vi "normalize.vi"(8 "error in":errorcluster caption="entrée d'erreur", 9 "X":string[][](array[string]), 10 "Type X":T1(ring), 11 "normalize":T3={"norm"="l2", "axis"=1, "copy"=TRUE, "Returns"="X"}) -> (0 "error out":errorcluster caption="sortie d'erreur", 3 "Data":T2)   [LabVIEW 2020]
uses:
  normalize.lvclass
panel:
  out "normalize.lvclass":refnum<class "normalize.lvclass">
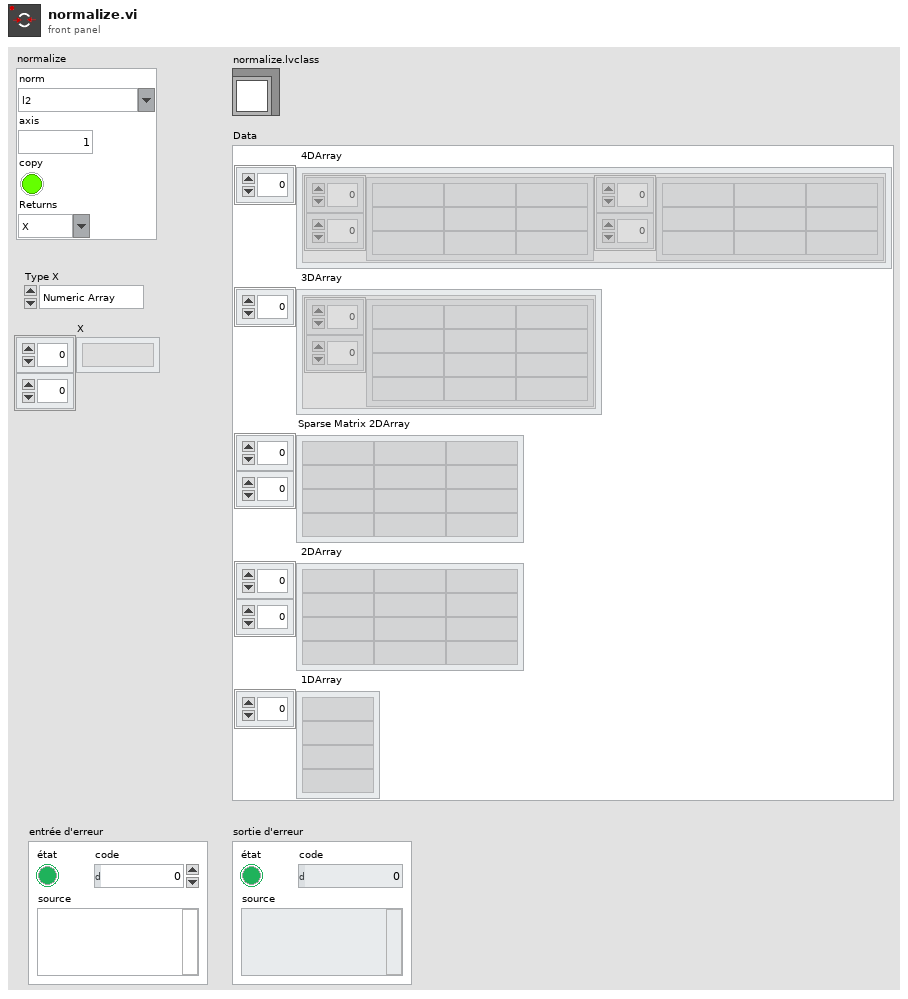
[diagram p1: front panel]
types:
  T1 = enum16{"Numeric Array", "String Array", "Sparse"}
  T2 = cluster{" 4DArray":cluster{"1":string[][], "2":string[][]}[], " 3DArray":cluster{"Tableau":string[][]}[], "Sparse Matrix 2DArray":string[][], " 2DArray":string[][], " 1DArray":string[]}
  T3 = cluster{"norm":string, "axis":i32, "copy":bool, "Returns":string}
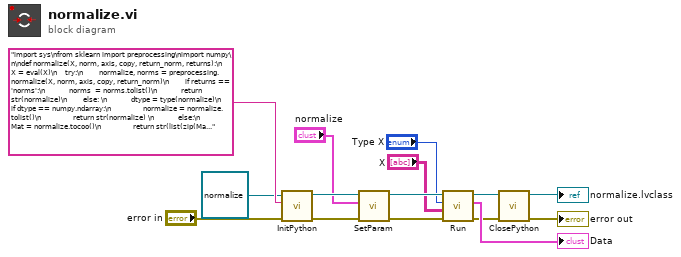
[diagram p0: block diagram]
diagram:
  n1 = call-dynamic "InitPython.vi"("error in (no error)"="error in", "Python Instruction"="import sys\nfrom sklearn import preprocessing\nimport numpy\n\ndef normalize(X, norm, axis, copy, return_norm, returns):\n    X = eval(X)\n    try:\n        normalize, norms = preprocessing.normalize(X, norm, axis, copy, return_norm)\n        if returns == 'norms':\n            norms  = norms.tolist()\n            return str(normalize)\n        else: \n            dtype = type(normalize)\n            if dtype == numpy.ndarray:\n                normalize = normalize.tolist()\n                return str(normalize) \n            else:\n                Mat = normalize.tocoo()\n                return str(list(zip(Mat.row, Mat.col, Mat.data)))\n    except:\n        erreur = sys.exc_info()\n        typerr = u\"%s\" % (erreur[0])\n        typerr = typerr[typerr.find(\"'\")+1:typerr.rfind(\"'\")]\n        msgerr = u\"%s\" % (erreur[1])\n        message = str('/!\\\\ {0} : {1}'. format(typerr,msgerr))\n        return message", "Scikit-learn en entrée"=refnum<class "normalize.lvclass"> refnum ("normalize.lvclass")) -> ("error out"=w10:errorcluster, "Scikit-learn en sortie"=w11:refnum<class "normalize.lvclass">)  [unwired: 7 in]
  n2 = call-dynamic "SetParam.vi"("error in (no error)"=w10, "normalize"="normalize", "normalize.lvclass"=w11) -> ("error out"=w6:errorcluster, "normalize.lvclass"=w8:refnum<class "normalize.lvclass">)  [unwired: 7 in]
  n3 = call-dynamic "Run.vi"("error in (no error)"=w6, "X"="X", "Type X"="Type X", "normalize.lvclass"=w8) -> ("error out"=w3:errorcluster, "Data"=→"Data":T2, "normalize.lvclass"=w5:refnum<class "normalize.lvclass">)  [unwired: 5 in]
  n4 = call-dynamic "ClosePython.vi"("error in (no error)"=w3, "Scikit-learn en entrée"=w5) -> ("error out"=→"error out":errorcluster, "Scikit-learn en sortie"=→"normalize.lvclass":refnum<class "normalize.lvclass">)  [unwired: 8 in]
